vi "ST example startup.vi"() -> ()   [LabVIEW 2009]
panel:
  out "Begin Complete":bool
  # "THIS IS THE INITIALIZATION ROUTINE FOR THE ST R17 ROBOT"
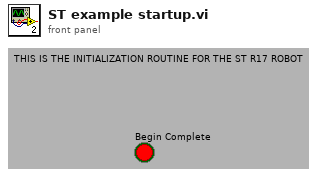
[diagram p1: front panel]
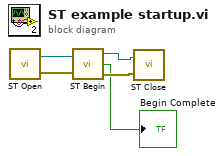
[diagram p0: block diagram]
diagram:
  n1 = call "ST Open.vi"() -> ("VISA resource name out"=w5:refnum<visa-resource-name>, "error out"=w4:errorcluster)  [unwired: 1 in]
  n2 = call "ST Begin.vi"("VISA resource name in"=w5, "error in"=w4) -> ("VISA resource name out"=w3:refnum<visa-resource-name>, "Begin Complete"=→"Begin Complete":bool, "error out"=w2:errorcluster)
  n3 = call "ST Close.vi"("error in (no error)"=w2, "VISA resource name"=w3) -> ()
